vi "Export_imageFileName.vi"(0 "ITC503 Current Values":T2 {"ITC503 Gradient" format="%.2f"; "ITC503 Setpoint" min=-273.0 max=300000.0 step=0.0001 format="%.1f"; "ITC503 I" format="%_1f"; "ITC503 P" format="%_1f"; "ITC503 Temperature" min=0.0 max=1645.0 step=1e-05 format="%.2f"; "ITC503 Heater" min=0.0 max=100.0 step=0.01 scale=0.0..100.0}, 1 "iHR Current Values":T3={"iHR 550 Front Entrance"=0.0, "iHR550 Side Exit"=0.0, "iHR550 Wavelength"=897.9988, "iHR550 Exit Mirror"=2, "iHR550 Grating"="1", "Grating Index"=1} {"iHR550 Exit Mirror" items=["EntranceMirror", "ExitMirror", "Front", "Side"]}, 2 "Spectra Settings":T1={"Integration Time"=10.0, "Repetitions"=10, "Mapping Spectra"=TRUE} caption="Mapping Spectra Settings" {"Repetitions" min=1 max=100 step=1; "Integration Time" min=0.5 max=6000.0 step=1.0 format="%.1f"}, 3 "Drive Current Values":T4 {"Position"."Drive Z Position" min=-273.0 max=300000.0 step=0.0001 format="%.1f"; "Position"."Drive Y Position" min=-273.0 max=300000.0 step=0.0001 format="%.1f"; "Position"."Drive X Position" min=-273.0 max=300000.0 step=0.0001 format="%.1f"; "Voltages"."Drive Z Voltage" min=-273.0 max=300000.0 step=0.0001 format="%.1f"; "Voltages"."Drive Y Voltage" min=-273.0 max=300000.0 step=0.0001 format="%.1f"; "Voltages"."Drive X Voltage" min=-273.0 max=300000.0 step=0.0001 format="%.1f"}, 4 "CCD3500 Temperature":dbl caption="Temp. (°C)" min=10.0 max=160.0 step=0.1 format="%.1f") -> (5 "Filename":string)   [LabVIEW 2010]
uses:
  ESA-C/TypeDefs/ESA-C Current Values.ctl
  iHR550/TypeDefs/iHR Current Values.ctl
  ITC503/TypeDefs/ITC503 Current Values.ctl
  Mapping/TypeDefs/Mapping Spectra Params.ctl
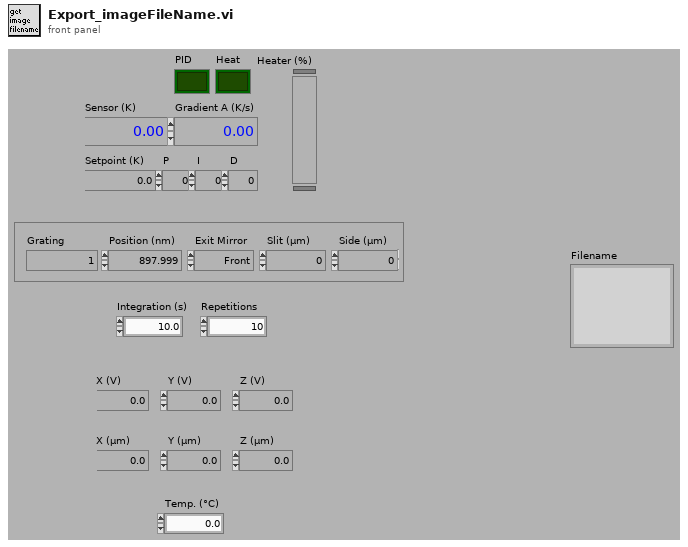
[diagram p1: front panel]
types:
  T1 = typedef "Mapping Spectra Params.ctl" = cluster{"Integration Time":dbl, "Repetitions":u16, "Mapping Spectra":bool}
  T2 = typedef "ITC503 Current Values.ctl" = cluster{"ITC503 Heater":dbl, "ITC503 Temperature":dbl, "ITC503 P":dbl, "ITC503 I":dbl, "ITC503 D":dbl, "ITC503 Setpoint":dbl, "ITC503 Gradient":dbl, "ITC503 Heater Auto":bool, "ITC503 PID Auto":bool}
  T3 = typedef "iHR Current Values.ctl" = cluster{"iHR 550 Front Entrance":dbl, "iHR550 Side Exit":dbl, "iHR550 Wavelength":dbl, "iHR550 Exit Mirror":i32, "iHR550 Grating":string, "Grating Index":i32}
  T4 = typedef "ESA-C Current Values.ctl" = cluster{"Voltages":cluster{"Drive X Voltage":dbl, "Drive Y Voltage":dbl, "Drive Z Voltage":dbl}, "Position":cluster{"Drive X Position":dbl, "Drive Y Position":dbl, "Drive Z Position":dbl}}
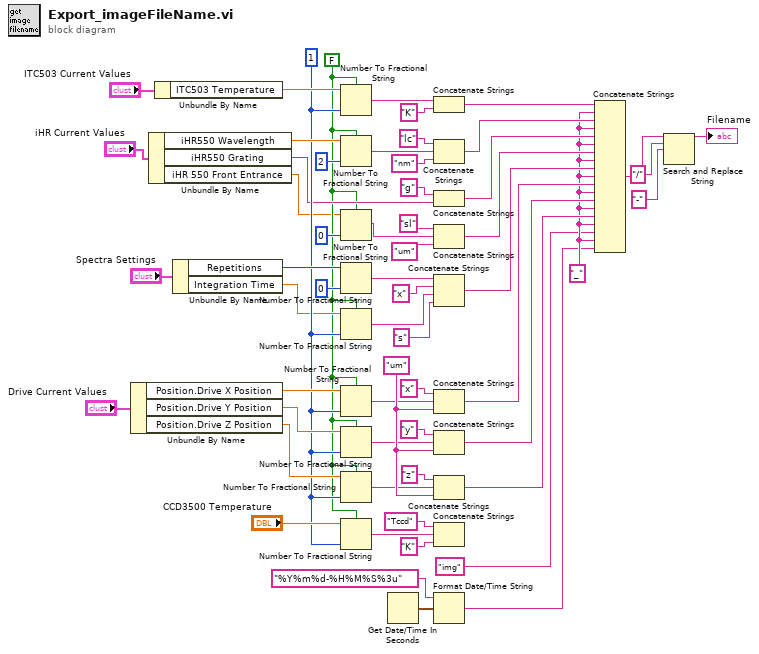
[diagram p0: block diagram]
diagram:
  w3 = "_" ("String")
  w33 = "um" ("String")
  w5 = FALSE ("Systemdezimalzeichen verwenden (T)")
  w47 = i16 1 ("Genauigkeit (6)")
  n1 = Unbundle By Name("Drive Current Values") -> ("Position.Drive X Position"=w53:dbl, "Position.Drive Y Position"=w52:dbl, "Position.Drive Z Position"=w51:dbl)
  n2 = Unbundle By Name("iHR Current Values") -> ("iHR550 Wavelength"=w50:dbl, "iHR550 Grating"=w25:string, "iHR 550 Front Entrance"=w4:dbl)
  n3 = Unbundle By Name("ITC503 Current Values") -> ("ITC503 Temperature"=w55:dbl)
  n4 = Unbundle By Name("Spectra Settings") -> ("Repetitions"=w54:u16, "Integration Time"=w39:dbl)
  n5 = Number To Fractional String(use system decimal point (T)=w5, number=w55, precision (6)=w47) -> (F-format string=w46:string)  [unwired: 1 in]
  n6 = Number To Fractional String(use system decimal point (T)=w5, number=w50, precision (6)=i16 2 ("Genauigkeit (6)")) -> (F-format string=w35:string)  [unwired: 1 in]
  n7 = Number To Fractional String(use system decimal point (T)=w5, number=w4, precision (6)=i16 0 ("Genauigkeit (6)")) -> (F-format string=w8:string)  [unwired: 1 in]
  n8 = Number To Fractional String(number=w54, precision (6)=i16 0 ("Genauigkeit (6)")) -> (F-format string=w42:string)  [unwired: 2 in]
  n9 = Number To Fractional String(use system decimal point (T)=w5, number=w39, precision (6)=w47) -> (F-format string=w41:string)  [unwired: 1 in]
  n10 = Number To Fractional String(use system decimal point (T)=w5, number=w53, precision (6)=w47) -> (F-format string=w32:string)  [unwired: 1 in]
  n11 = Number To Fractional String(use system decimal point (T)=w5, number=w52, precision (6)=w47) -> (F-format string=w31:string)  [unwired: 1 in]
  n12 = Number To Fractional String(use system decimal point (T)=w5, number=w51, precision (6)=w47) -> (F-format string=w30:string)  [unwired: 1 in]
  n13 = Number To Fractional String(use system decimal point (T)=w5, number="CCD3500 Temperature", precision (6)=w47) -> (F-format string=w38:string)  [unwired: 1 in]
  n14 = Get Date/Time In Seconds() -> (seconds since 1Jan1904=w13:timestamp)
  n15 = Concatenate Strings(w46, "K" ("String")) -> (w24:string)
  n16 = Concatenate Strings("lc" ("String"), w35, "nm" ("String")) -> (w23:string)
  n17 = Concatenate Strings("g" ("String"), w25) -> (w22:string)
  n18 = Concatenate Strings("sl" ("String"), w8, "um" ("String")) -> (w7:string)
  n19 = Concatenate Strings(w42, "x" ("String"), w41, "s" ("String")) -> (w6:string)
  n20 = Concatenate Strings("x" ("String"), w32, w33) -> (w21:string)
  n21 = Concatenate Strings("y" ("String"), w31, w33) -> (w20:string)
  n22 = Concatenate Strings("z" ("String"), w30, w33) -> (w19:string)
  n23 = Concatenate Strings("Tccd" ("String"), w38, "K" ("String")) -> ()  [unwired: 1 out]
  n24 = Format Date/Time String(time format string (%c)="%Y%m%d-%H%M%S%3u", seconds (now)=w13) -> (date/time string=w2:string)  [unwired: 1 in]
  n25 = Concatenate Strings(w24, w3, w23, w3, w22, w3, w7, w3, w6, w3, w21, w3, w20, w3, w19, w3, "img" ("string"), w3, w2) -> (w17:string)
  n26 = Search and Replace String(input string=w17, search string="/" ("Such-String"), replace string="-" ("replace string (\"\")")) -> (result string=→"Filename":string)  [unwired: 5 in, 3 out]
